vi "Write Box ItemNames.vi"(8 "error in (no error)":errorcluster, 11 "BetterListboxHandle in":refnum<class "BetterListboxHandle.lvclass">) -> (0 "error out":errorcluster, 3 "BetterListboxHandle out":refnum<class "BetterListboxHandle.lvclass">)   [LabVIEW 2020, in "BetterDragAndDrop.lvlib" / "BetterListboxHandle.lvclass"]
uses:
  BetterListboxHandle.lvclass
  C:/DSCE code/Open-source/betterdraganddrop_GIT/Source/Classes/BetterHandle/BetterHandle.lvclass
  BetterHandle/BetterHandle.lvclass/BetterHandle.ctl
  BetterListboxHandle.lvclass/BetterListboxHandle.ctl
  BetterTreeItem/BetterItem.lvclass
  BetterHandle/BetterHandle.lvclass
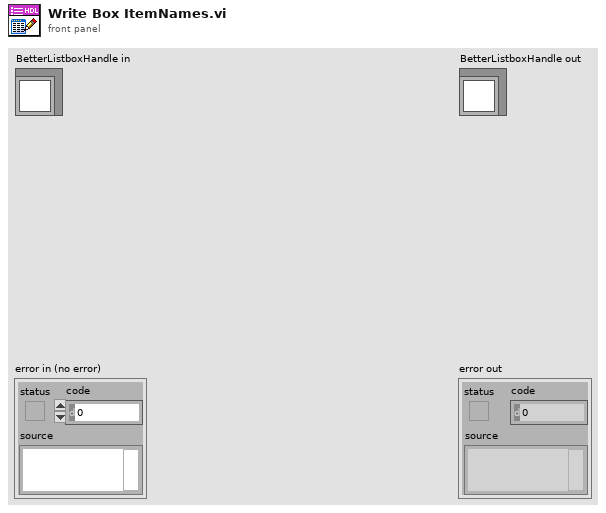
[diagram p1: front panel]
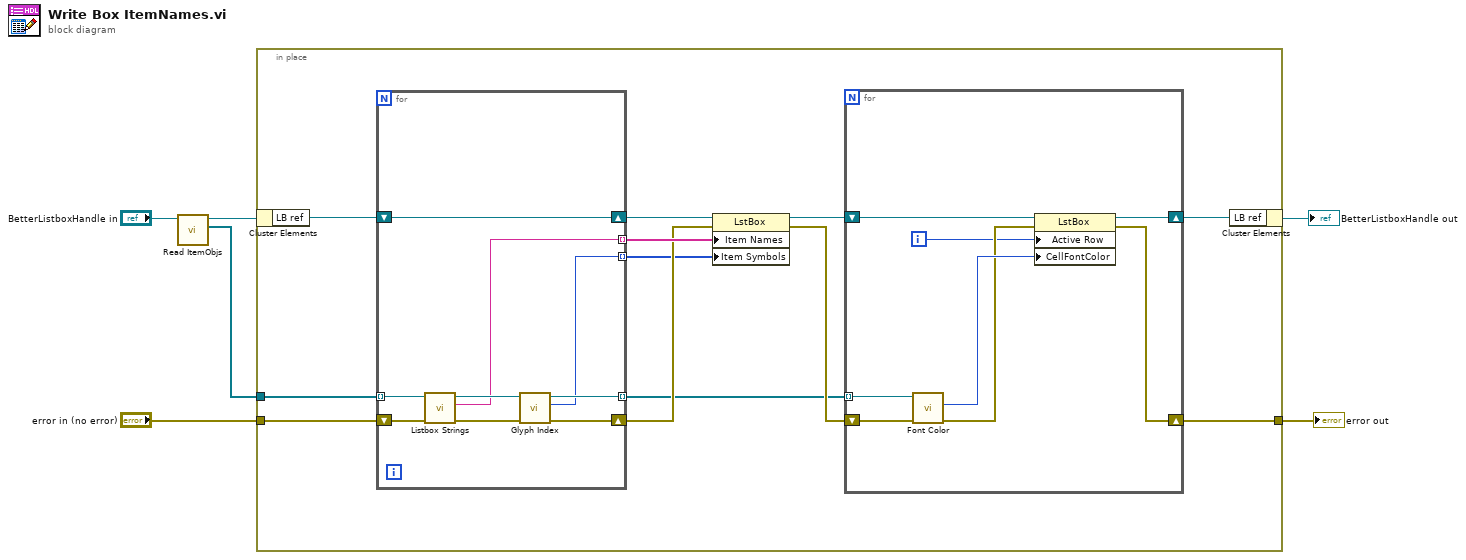
[diagram p0: block diagram]
diagram:
  n1 = call "Read ItemObjs.vi"("BetterHandle in"="BetterListboxHandle in") -> ("ItemObjs"=w5:refnum<class "BetterItem.lvclass">[], "BetterHandle out"=w6:refnum<class "BetterListboxHandle.lvclass">)  [unwired: 9 in]
  n2 = in-place {
    in-place-border: w5 -> [w18]
    in-place-border: "error in (no error)" -> [w16]
    in-place-border: [w9] -> w1
    n3 = in-place-cluster #1(w6) -> ("LB ref"=w8:refnum<vi>)
    n4 = for {
      tunnel: w18 -> [w31] mode=indexing
      tunnel: [w28] -> w17 mode=indexing
      shift-right: [w34] -> w15
      shift-left: w16 -> [w30]
      tunnel: [w35] -> w12 mode=indexing
      tunnel: [w33] -> w11 mode=indexing
      shift-right: [w32] -> w7
      shift-left: w8 -> [w32]
      n5 = call-dynamic "Listbox Strings.vi"("error in (no error)"=w30, "BetterItem in"=w31) -> ("error out"=w27:errorcluster, "ItemName"=w28:string, "BetterItem out"=w29:refnum<class "BetterItem.lvclass">)  [unwired: 7 in]
      n6 = call-dynamic "Glyph Index.vi"("error in (no error)"=w27, "BetterItem in"=w29) -> ("error out"=w34:errorcluster, "Glyph Index"=w33:i32, "BetterItem out"=w35:refnum<class "BetterItem.lvclass">)  [unwired: 7 in]
    }
    n7 = property class="LstBox"(reference=w7, error in=w15, "Item Names"=w17, "Item Symbols"=w11) -> (reference out=w14:refnum<vi>, error out=w13:errorcluster)
    n8 = for {
      shift-right: [w23] -> w10
      shift-left: w14 -> [w26]
      shift-right: [w22] -> w9
      shift-left: w13 -> [w21]
      tunnel: w12 -> [w25] mode=indexing
      i -> [w19]
      n9 = call-dynamic "Font Color.vi"("error in (no error)"=w21, "BetterItem in"=w25) -> ("error out"=w20:errorcluster, "Font Color"=w24:u32)  [unwired: 7 in, 1 out]
      n10 = property class="LstBox"(reference=w26, error in=w20, "Active Row"=w19, "CellFontColor"=w24) -> (reference out=w23:refnum<vi>, error out=w22:errorcluster)
    }
    n11 = in-place-cluster #1("LB ref"=w10) -> (→"BetterListboxHandle out":refnum<class "BetterListboxHandle.lvclass">)
  }
  "error out" <- w1
